vi "Frame Conversion Test.vi"() -> ()   [LabVIEW 2018]
uses:
  Classes/Video File/Video File.lvclass
  Classes/Video Frame/Video Frame.lvclass
panel:
  out "Depth Values 2":dbl[](array[numeric])
  out "Depth Values":dbl[](array[numeric])
  out "Image ROI":T1(plugin-control)
  out "error out":errorcluster
  out "Image":T1(plugin-control)
  in  "Path":path
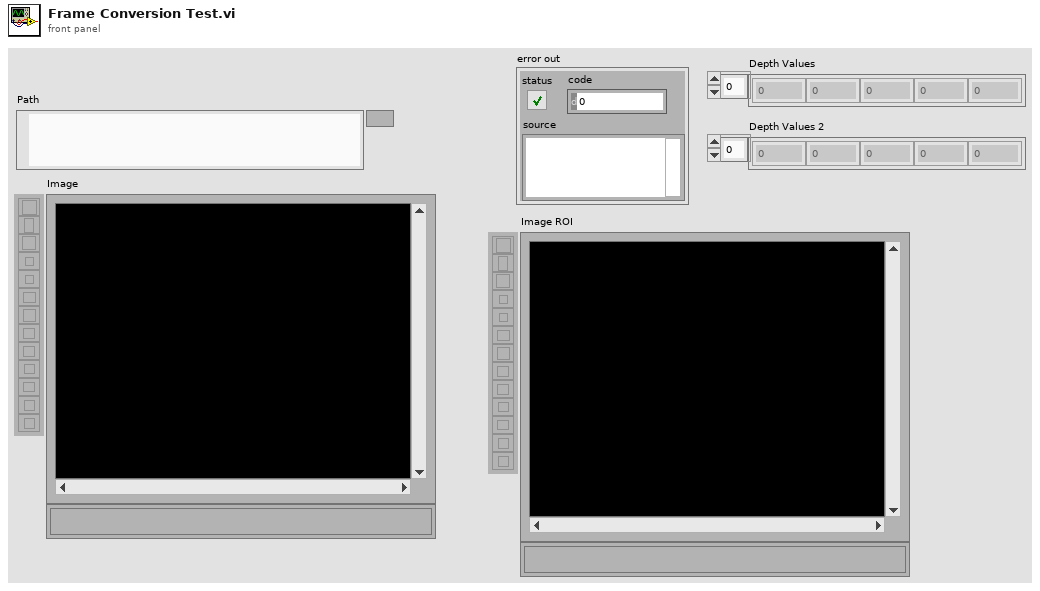
[diagram p1: front panel]
types:
  T1 = typedef "IMAQ Image.ctl" = refnum<image>
  T2 = cluster{"Global Rectangle":i32[], "Contours":cluster{"Contour Type":u32, "ROI Type":u32, "Points":i32[]}[]}
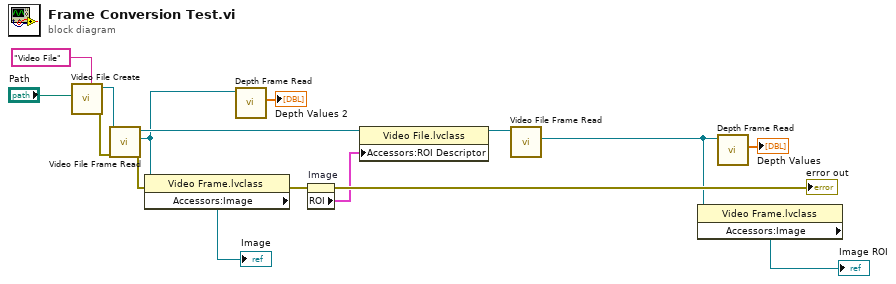
[diagram p0: block diagram]
diagram:
  n1 = call "Video File Create.vi"("Identifier"="Video File", "Video Path (\"\")"="Path") -> ("error out"=w12:errorcluster, "Video File out"=w14:refnum<class "Video File.lvclass">)  [unwired: 8 in]
  n2 = call-dynamic "Video File Frame Read.vi"("error in (no error)"=w12, "Video File in"=w14) -> ("error out"=w11:errorcluster, "Video Frame out"=w2:refnum<class "Video Frame.lvclass">, "Video File out"=w6:refnum<class "Video File.lvclass">)  [unwired: 5 in, 2 out]
  n3 = property class="Video Frame.lvclass"(reference=w2, error in=w11) -> (error out=w10:errorcluster, "Accessors:Image"=→"Image":T1)  [unwired: 1 out]
  n4 = call-dynamic "Depth Frame Read.vi"("Video Frame in"=w2) -> ("Depth Values"=→"Depth Values 2":dbl[])  [unwired: 6 in, 4 out]
  n5 = property on="Image" class="ImageControl"(error in=w10) -> (error out=→"error out":errorcluster, "ROI"=w5:T2)  [unwired: 1 in, 1 out]
  n6 = property class="Video File.lvclass"(reference=w6, "Accessors:ROI Descriptor"=w5) -> (reference out=w4:refnum<class "Video File.lvclass">)  [unwired: 1 in, 1 out]
  n7 = call-dynamic "Video File Frame Read.vi"("Video File in"=w4) -> ("Video Frame out"=w3:refnum<class "Video Frame.lvclass">)  [unwired: 6 in, 4 out]
  n8 = property class="Video Frame.lvclass"(reference=w3) -> ("Accessors:Image"=→"Image ROI":T1)  [unwired: 1 in, 2 out]
  n9 = call-dynamic "Depth Frame Read.vi"("Video Frame in"=w3) -> ("Depth Values"=→"Depth Values":dbl[])  [unwired: 6 in, 4 out]
